vi "RemoveNamedSemaphorePrefix.vi"(10 "Name In":string) -> (2 "Name Out":string)   [LabVIEW 2020]
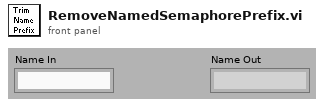
[diagram p1: front panel]
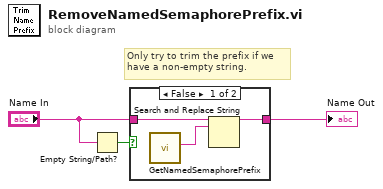
[diagram p0: block diagram]
diagram:
  # "Only try to trim the prefix if we\nhave a non-empty string."
  n1 = Empty String/Path?(string/path="Name In") -> (empty?=w3:bool)
  n2 = case shown="False" w3 {
    tunnel: "Name In" -> [w6 w7]
    tunnel: [w5 w7] -> w2
    frame False {
      n3 = call "GetNamedSemaphorePrefix.vi"() -> ("Named Semaphore Prefix"=w4:string)  [unwired: 11 out]
      n4 = Search and Replace String(input string=w6, search string=w4) -> (result string=w5:string)  [unwired: 1 in, 8 out]
    }
    frame True {
    }
  }
  "Name Out" <- w2
